vi "Laser Power Scaling.vi"(4 "Boolean":bool, 6 "Stream Exposure Time (ms)":dbl, 7 "Laser Power (mW)":dbl, 9 "Excitation":T1, 10 "Live Exposure Time (ms)":dbl, 11 "Message Enqueuer in":refnum<class "Message Enqueuer.lvclass">) -> (3 "Message Enqueuer out":refnum<class "Message Enqueuer.lvclass">)   [LabVIEW 2018]
uses:
  Resources/Type Defs/Excitation.ctl
  <vilib>/ActorFramework/Message Enqueuer/Message Enqueuer.lvclass
  Application Messages/Set Laser Power Msg/Set Laser Power Msg.lvclass/Set Laser Power Msg.ctl
  <vilib>/ActorFramework/Message Enqueuer/Message Enqueuer.lvclass/Message Enqueuer.ctl
  <vilib>/ActorFramework/Message Enqueuer/Enqueue.vi
  Application Messages/Set Laser Power Msg/Set Laser Power Msg.lvclass
  C:/Program Files/National Instruments/LabVIEW 2018/vi.lib/ActorFramework/Message/Message.lvclass
  <vilib>/ActorFramework/Message Priority Queue/Priority Enqueue.vi
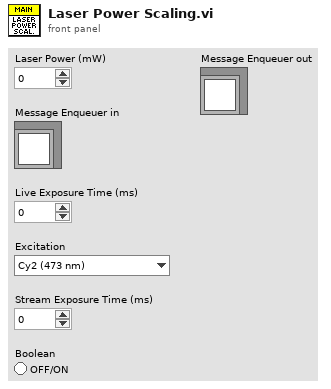
[diagram p1: front panel]
types:
  T1 = typedef "Excitation.ctl" = enum16{"Cy2 (473 nm)", "Cy3 (532 nm)", "Cy5 (639 nm)", "Cy7 (730 nm)", "Cy2/Cy3", "Cy3/Cy5", "Cy3/Cy7", "Cy5/Cy7"}
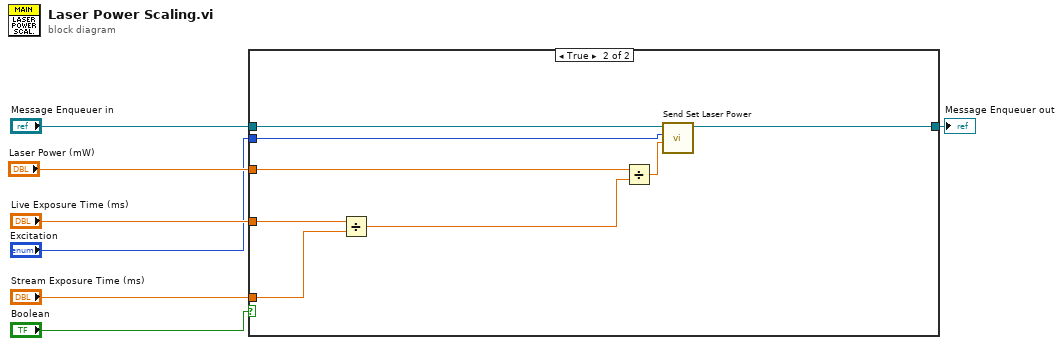
[diagram p0: block diagram]
diagram:
  n1 = case shown="True" "Boolean" {
    tunnel: "Excitation" -> [_ w15]
    tunnel: "Live Exposure Time (ms)" -> [_ w14]
    tunnel: "Stream Exposure Time (ms)" -> [_ w13]
    tunnel: "Message Enqueuer in" -> [w8 w12]
    tunnel: [w8 w9] -> w3
    tunnel: "Laser Power (mW)" -> [_ w11]
    frame False {
    }
    frame True {
      n2 = Divide(x=w14, y=w13) -> (x/y=w16:dbl)
      n3 = Divide(x=w11, y=w16) -> (x/y=w10:dbl)
      n4 = call "Send Set Laser Power.vi"("Power"=w10, "Wavelength"=w15, "Message Enqueuer"=w12) -> ("Message Enqueuer out"=w9:refnum<class "Message Enqueuer.lvclass">)  [unwired: 7 in, 1 out]
    }
  }
  "Message Enqueuer out" <- w3
